vi "Get LakeShore 340 Mode.vi"(8 "error in (no error)":errorcluster, 10 "Output #":i32=1, 11 "VISA Resource Name":refnum<visa-resource-name>) -> (0 "error out":errorcluster, 1 "on/off":i32, 2 "Lake shore mode":T1, 3 "VISA Resource Name Out":refnum<visa-resource-name>, 5 "Input chan":string, 6 "powerup enable":i32, 7 "units":i32)   [LabVIEW 2021]
uses:
  LakeShore340 Mode.ctl
  GPIB/VISA  Send Receive.vi
  Simple VISA Reader/Simple VISA Reader Driver.lvclass
panel:
  out "data string out 2":string
  out "data string out":string
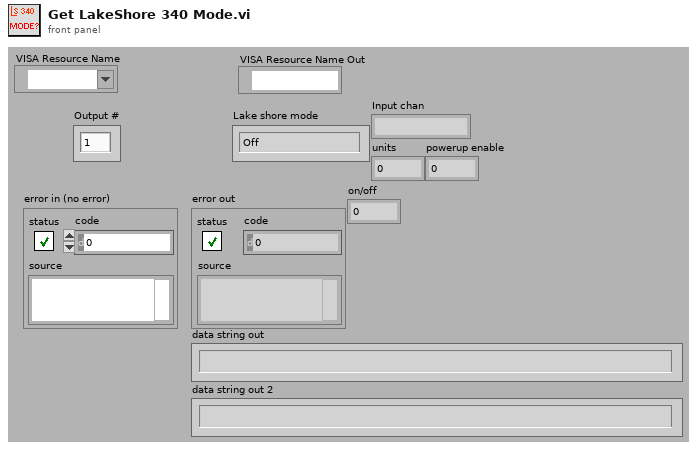
[diagram p1: front panel]
types:
  T1 = typedef "LakeShore340 Mode.ctl" = enum16{"Off", "Manual PID", "Zone", "Open loop", "AutoTune PID", "AutoTune PI", "AutoTune P"}
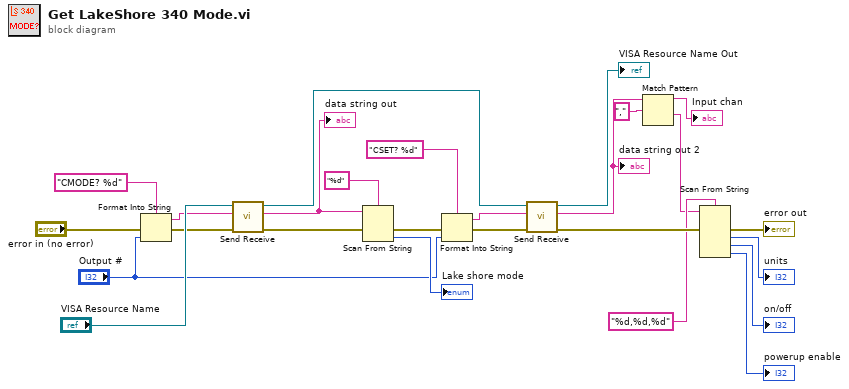
[diagram p0: block diagram]
diagram:
  n1 = Format Into String(format string="CMODE? %d" ("data string"), error in="error in (no error)", "Output #") -> (resulting string=w22:string, error out=w24:errorcluster)  [unwired: 1 in]
  n2 = call-poly "Send Receive.vi"("error in (no error)"=w24, "data string in"=w22, "VISA Resource Name"="VISA Resource Name") -> ("error out"=w19:errorcluster, "data string out"=w21:string, "VISA Resource Name Out"=w14:refnum<visa-resource-name>)  [unwired: 6 in]
  "data string out" <- w21
  n3 = Scan From String(format string="%d", input string=w21, error in=w19) -> (error out=w17:errorcluster, output 1=→"Lake shore mode":T1)  [unwired: 2 in, 2 out]
  n4 = Format Into String(format string="CSET? %d" ("data string"), error in=w17, "Output #") -> (resulting string=w12:string, error out=w16:errorcluster)  [unwired: 1 in]
  n5 = call-poly "Send Receive.vi"("error in (no error)"=w16, "data string in"=w12, "VISA Resource Name"=w14) -> ("error out"=w10:errorcluster, "data string out"=w6:string, "VISA Resource Name Out"=→"VISA Resource Name Out":refnum<visa-resource-name>)  [unwired: 6 in]
  "data string out 2" <- w6
  n6 = Match Pattern(string=w6, regular expression=",") -> (before substring=→"Input chan":string, after substring=w4:string)  [unwired: 1 in, 2 out]
  n7 = Scan From String(format string="%d,%d,%d", input string=w4, error in=w10) -> (error out=→"error out":errorcluster, output 1=→"units":i32, output 2=→"on/off":i32, output 3=→"powerup enable":i32)  [unwired: 4 in, 2 out]
